vi "Shortest Distance Absolute.vi"(1 "Current Angle":dbl(knob)=41.7137932364482 scale=0.0..360.0, 3 "Set Point":dbl(knob)=41.7137932364482 scale=0.0..360.0) -> (7 "Better Angle":dbl(knob)=41.7137932364482 scale=0.0..360.0, 9 "Degres To Travel":dbl)   [LabVIEW 2018]
uses:
  <vilib>/Analysis/coordinate.llb/Angle Units.ctl
  <vilib>/Analysis/coordinate.llb/Angle Range (Degree).ctl
  <vilib>/Analysis/coordinate.llb/Wrap Angle (scalar).vi
  <vilib>/Analysis/NI_AAL_Angle.lvlib
panel:
  out "case select":dbl
  out "s? t:f":dbl
  out "abs(x)":dbl
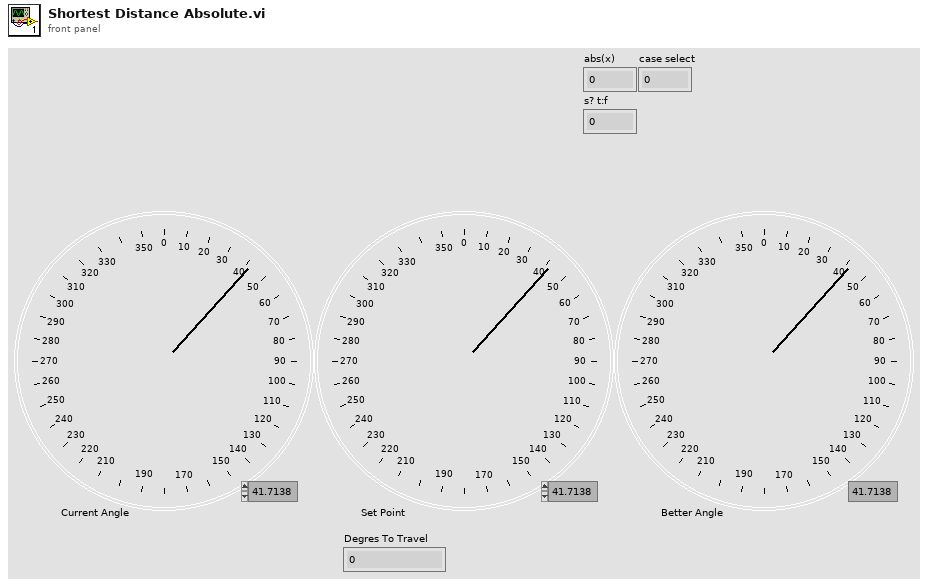
[diagram p1: front panel]
types:
  T1 = typedef "NI_AAL_Angle.lvlib/Angle Range (Degree).ctl" = u16
  T2 = typedef "NI_AAL_Angle.lvlib/Angle Units.ctl" = i32
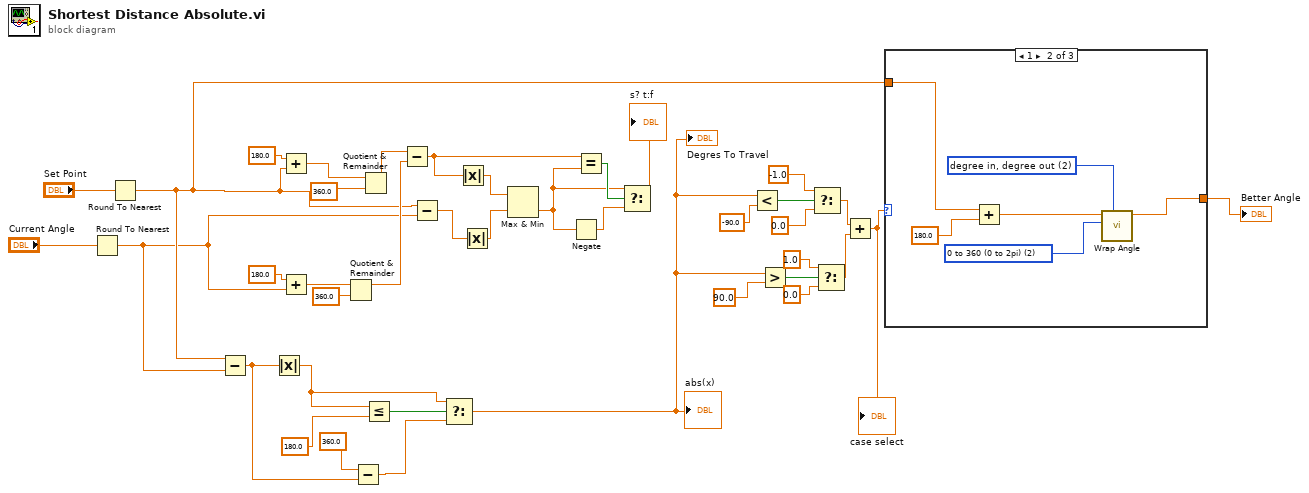
[diagram p0: block diagram]
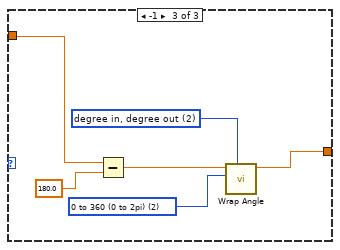
[diagram p3: hidden frame]
diagram:
  n1 = Round To Nearest(number="Current Angle") -> (nearest integer value=w1:dbl)
  n2 = Round To Nearest(number="Set Point") -> (nearest integer value=w2:dbl)
  n3 = Subtract(x=w2, y=w1) -> (x-y=w5:dbl)
  n4 = Absolute Value(x=w5) -> (abs(x)=w6:dbl)
  n5 = Add(x=180.0, y=w2) -> (x+y=w34:dbl)
  n6 = Add(x=180.0, y=w1) -> (x+y=w37:dbl)
  n7 = Quotient & Remainder(x=w37, y=360.0) -> (x-y*floor(x/y)=w28:dbl)  [unwired: 1 out]
  n8 = Subtract(x=360.0, y=w5) -> (x-y=w7:dbl)
  n9 = Quotient & Remainder(x=w34, y=360.0) -> (x-y*floor(x/y)=w29:dbl)  [unwired: 1 out]
  n10 = Less Or Equal?(x=w6, y=180.0 ("x")) -> (x <= y?=w8:bool)
  n11 = Subtract(x=w29, y=w28) -> (x-y=w27:dbl)
  n12 = Subtract(x=w2, y=w1) -> (x-y=w32:dbl)
  n13 = Select(t=w6, s=w8, f=w7) -> (s? t:f=w3:dbl)
  "Degres To Travel" <- w3
  "abs(x)" <- w3
  n14 = Absolute Value(x=w27) -> (abs(x)=w30:dbl)
  n15 = Absolute Value(x=w32) -> (abs(x)=w31:dbl)
  n16 = Max & Min(x=w30, y=w31) -> (min(x,y)=w25:dbl)  [unwired: 1 out]
  n17 = Negate(x=w25) -> (-x=w26:dbl)
  n18 = Equal?(x=w27, y=w25) -> (x = y?=w39:bool)
  n19 = Select(t=w25, s=w39, f=w26) -> (s? t:f=→"s? t:f":dbl)
  n20 = Less?(x=w3, y=-90.0 ("lower limit")) -> (x < y?=w19:bool)
  n21 = Greater?(x=w3, y=90.0 ("upper limit")) -> (0:w21:bool)
  n22 = Select(t=-1.0, s=w19, f=0.0) -> (s? t:f=w12:dbl)
  n23 = Select(t=1.0, s=w21, f=0.0) -> (s? t:f=w11:dbl)
  n24 = Add(x=w12, y=w11) -> (x+y=w13:dbl)
  "case select" <- w13
  n25 = case shown="1" w13 {
    tunnel: w2 -> [w40 w42 w48]
    tunnel: [w40 w41 w47] -> w14
    frame 0, Default {
    }
    frame 1 {
      w45 = T1 2 items=["none", "-180 to 180 (-pi to pi)", "0 to 360 (0 to 2pi)"] ("angle range")
      w46 = T2 2 items=["radian in, radian out", "radian in, degree out", "degree in, degree out", "degree in, radian out"] ("angle units")
      n26 = Add(x=w42, y=180.0) -> (x+y=w43:dbl)
      n27 = call-poly <vilib>:"Wrap Angle.vi"("angle units"=w46, "angle range"=w45, "angle in"=w43) -> ("angle out"=w41:dbl)  [unwired: 7 in, 1 out]
    }
    frame -1 {
      w51 = T1 2 items=["none", "-180 to 180 (-pi to pi)", "0 to 360 (0 to 2pi)"] ("angle range")
      w52 = T2 2 items=["radian in, radian out", "radian in, degree out", "degree in, degree out", "degree in, radian out"] ("angle units")
      n28 = Subtract(x=w48, y=180.0) -> (x-y=w49:dbl)
      n29 = call-poly <vilib>:"Wrap Angle.vi"("angle units"=w52, "angle range"=w51, "angle in"=w49) -> ("angle out"=w47:dbl)  [unwired: 7 in, 1 out]
    }
  }
  "Better Angle" <- w14
